vi "Detect expert based hardwares.vi"(11 "Expert name":string) -> (0 "error out":errorcluster, 2 "Product names":string[](array[string]), 3 "Alias names":string[](array[string]))   [LabVIEW 2021]
uses:
  <vilib>/nisyscfg/Close (System).vi
  <vilib>/nisyscfg/nisyscfg.lvlib
  <resource>/objmgr/niMIDebugSession.rc
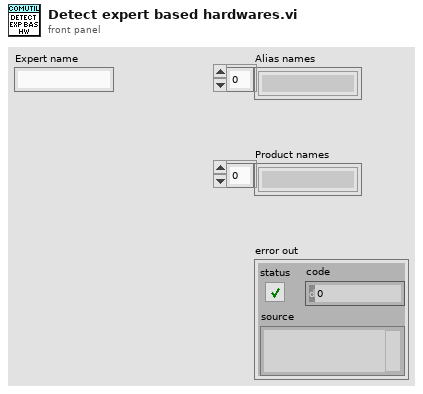
[diagram p1: front panel]
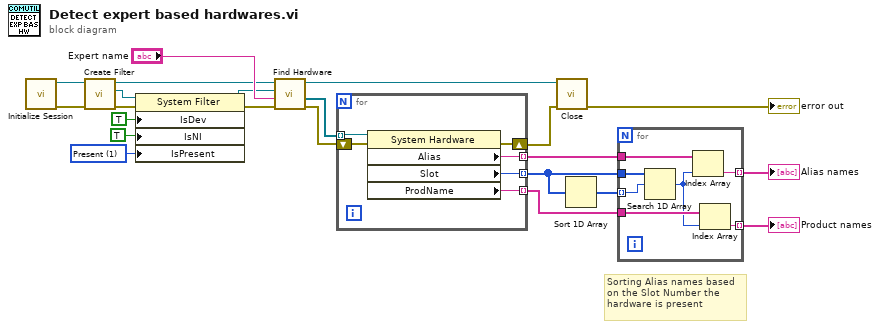
[diagram p0: block diagram]
diagram:
  w7 = 1 items=["Initializing"=-2, "Unknown"=-1, "Not Present"=0, "Present"=1] ("Devices & Chassis:Is Present")
  # "Sorting Alias names based\non the Slot Number the \nhardware is present"
  n1 = call <vilib>:"Initialize Session.vi"() -> ("error out"=w15:errorcluster, "Session out"=w18:refnum<k21>)  [unwired: 10 in]
  n2 = call <vilib>:"Create Filter.vi"("error in (no error)"=w15, "Session in"=w18) -> ("error out"=w17:errorcluster, "Filter out"=w16:refnum<k20>, "Session out"=w11:refnum<k21>)  [unwired: 7 in]
  n3 = property class="System Filter"(reference=w16, error in=w17, "IsDev"=TRUE ("Is Device"), "IsNI"=TRUE ("Devices & Chassis:Is NI Product"), "IsPresent"=w7) -> (reference out=w10:refnum<k20>, error out=w12:errorcluster)
  n4 = call <vilib>:"Find Hardware.vi"("error in (no error)"=w12, "Experts"="Expert name", "Filter in"=w10, "Session in"=w11) -> ("error out"=w20:errorcluster, "Resources out"=w21:refnum<k20>[], "Session out"=w8:refnum<k21>)  [unwired: 4 in, 1 out]
  n5 = for {
    tunnel: w21 -> [w28] mode=indexing
    tunnel: [w25] -> w5 mode=indexing
    shift-right: [w26] -> w9
    shift-left: w20 -> [w27]
    tunnel: [w24] -> w4 mode=indexing
    tunnel: [w23] -> w2 mode=indexing
    n6 = property class="System Hardware"(reference=w28, error in=w27) -> (error out=w26:errorcluster, "Alias"=w25:string, "Slot"=w24:i32, "ProdName"=w23:string)  [unwired: 1 out]
  }
  n7 = call-poly <vilib>:"Close.vi"("error in (no error)"=w9, "Session in"=w8) -> ("error out"=→"error out":errorcluster)  [unwired: 9 in]
  n8 = Sort 1D Array(array=w4) -> (sorted array=w6:i32[])
  n9 = for {
    tunnel: w6 -> [w33] mode=indexing
    tunnel: w5 -> [w35]
    tunnel: w4 -> [w34]
    tunnel: [w32] -> w3 mode=indexing
    tunnel: w2 -> [w31]
    tunnel: [w29] -> w1 mode=indexing
    n10 = Search 1D Array(1D array=w34, element=w33) -> (index of element=w30:i32)  [unwired: 1 in]
    n11 = Index Array(array=w35, index=w30) -> (element=w32:string)
    n12 = Index Array(array=w31, index=w30) -> (element=w29:string)
  }
  "Alias names" <- w3
  "Product names" <- w1
